vi "LV8_10b.vi"() -> ()   [LabVIEW 2011]
uses:
  <vilib>/imath/engines/lvmath2/RunTimeEngine/ErrorHandling/NIMS_Finalize Error.vi
  <vilib>/imath/engines/lvmath2/RunTimeEngine/NodeEndStatement/NIMS_NodeEndStatement_Output.vi
  <instcachedir>/0/NIMS_NodeEndStatement_Output_53EC0D466D134D7ABD903AC30B43404B.lvgen/NIMS_NodeEndStatement_Output_53EC0D466D134D7ABD903AC30B43404B_000.vi
  <instcachedir>/0/NIMS_NodeEndStatement_Output_53EC0D466D134D7ABD903AC30B43404B.lvgen/NIMS_NodeEndStatement_Output_53EC0D466D134D7ABD903AC30B43404B_005.vi
  <vilib>/imath/engines/lvmath2/RunTimeEngine/RangeToken/NIMS_Range.vi
  <instcachedir>/0/NIMS_Range_0B7635FB69F84E19AA68E7FF959DF37C.lvgen/NIMS_Range_0B7635FB69F84E19AA68E7FF959DF37C_001.vi
  <vilib>/imathl/engines/lvmath/Functions/Error Handling/Create Error.vi
  <vilib>/imath/engines/lvmath2/RunTimeEngine/ArithmeticOperatorToken/NIMS_ArithmeticOperator_times.vi
  <instcachedir>/0/NIMS_ArithmeticOperator_times_3FA9DDB491BD45F6905798C0465C9825.lvgen/NIMS_ArithmeticOperator_times_3FA9DDB491BD45F6905798C0465C9825_000.vi
  <vilib>/imath/engines/lvmath2/RunTimeEngine/BuiltInFunctions/fft/NIMS_fft(GV).vi
  <instcachedir>/0/NIMS_fft(GV)_4C6467FC22F84E4BA42517A07EF978B0.lvgen/NIMS_fft(GV)_4C6467FC22F84E4BA42517A07EF978B0_001.vi
  <vilib>/imath/engines/lvmath2/RunTimeEngine/BuiltInFunctions/abs/NIMS_abs(signed).vi
  <instcachedir>/0/NIMS_abs(signed)_C4FCB8E6058B49B797C7C8D53CA5F6EC.lvgen/NIMS_abs(signed)_C4FCB8E6058B49B797C7C8D53CA5F6EC_006.vi
  <vilib>/imath/engines/lvmath2/RunTimeEngine/BuiltInFunctions/fftshift/NIMS_fftshift(GV).vi
  <instcachedir>/0/NIMS_fftshift(GV)_BD7A7BA9CA6B470B9A9F73A6A3FEEB3E.lvgen/NIMS_fftshift(GV)_BD7A7BA9CA6B470B9A9F73A6A3FEEB3E_001.vi
  <vilib>/imath/engines/lvmath2/RunTimeEngine/ErrorHandling/NIMS_Error From Error Code.vi
  <vilib>/imath/engines/lvmath2/RunTimeEngine/VariableToken/Read/NIMS_Get Elements - RV(_) - Check.vi
  <instcachedir>/0/NIMS_Get Elements - RV(_) - Check_B511B9D8E05044FE80F9F088FE24B20C.lvgen/NIMS_Get Elements - RV(_) - Check_B511B9D8E05044FE80F9F088FE24B20C_000.vi
  <vilib>/imath/engines/lvmath2/RunTimeEngine/BuiltInFunctions/linramp/NIMS_linramp.vi
  <vilib>/imath/engines/lvmath2/RunTimeEngine/ErrorHandling/NIMS_Create Error From Enums.vi
panel:
  in  "stop":bool
  in  "Fmax":dbl(slide)=0.6 scale=0.5..1.0
  in  "Tmax":dbl(slide)=4.0 scale=4.0..10.0
  out "Time Domain":cluster{"f":dbl[], "FX":dbl[]}[](graph)=[{"f"=[-4.0, -3.1666666666666665, -2.333333333333333, -1.5, -0.6666666666666665, 0.16666666666666696, 1.0, 1.833333333333334, 2.666666666666667], "FX"=[0.00013383022576488537, 0.0026509759544301056, 0.026221889093709518, 0.12951759566589174, 0.3194480055223523, 0.3934397161019399, 0.24197072451914337, 0.074311163558993, 0.011395986023797433]}, {"f"=array[2000 elements], "FX"=array[2000 elements]}]
  out "Frequency Domain":cluster{"f":dbl[], "FX":dbl[]}[](graph)=[{"f"=[-0.6, -0.475, -0.35, -0.22499999999999998, -0.09999999999999998, 0.025000000000000022, 0.15000000000000002, 0.275, 0.4], "FX"=[0.0008200746635147077, 0.011635913339555859, 0.08909490952726896, 0.3681379872984424, 0.82086871741554, 0.9877387833616438, 0.6413806259551537, 0.22474751427102416, 0.04249905628536254]}, {"f"=array[2000 elements], "FX"=array[2000 elements]}]
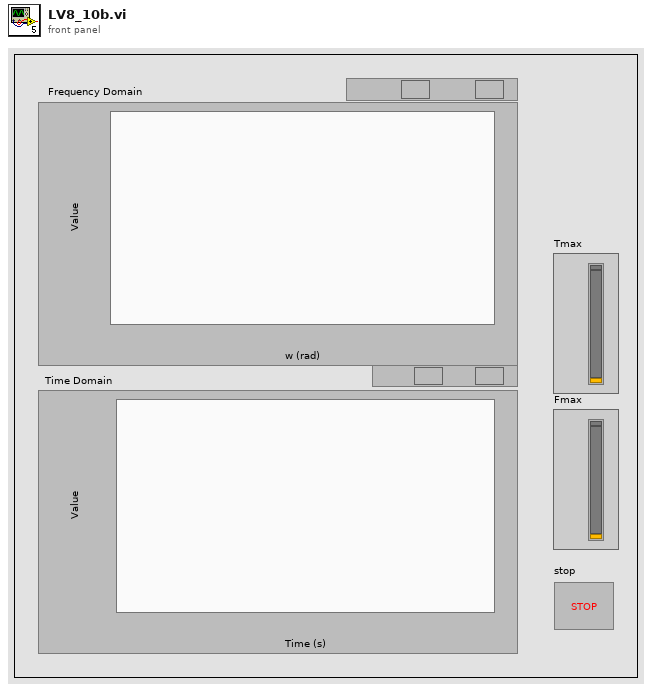
[diagram p1: front panel]
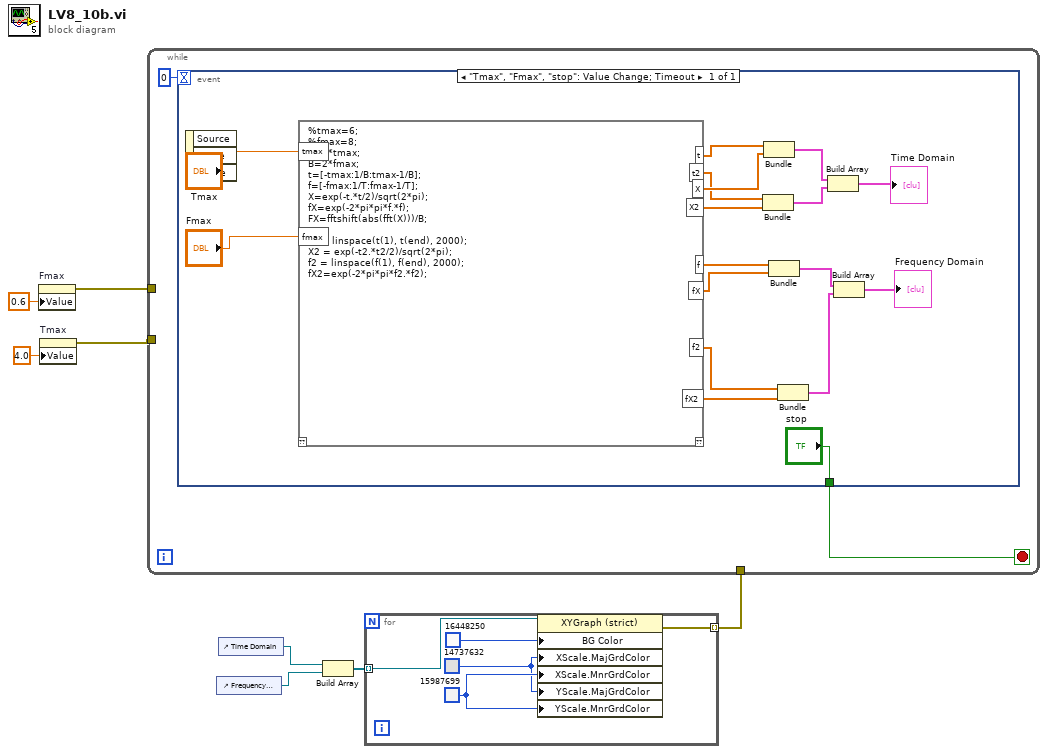
[diagram p0: block diagram]
diagram:
  n1 = property on="Fmax" class="Slide (strict)"("Value"=0.6 ("Fmax")) -> (error out=w6:errorcluster)  [unwired: 2 in, 1 out]
  n2 = property on="Tmax" class="Slide (strict)"("Value"=4.0 ("Tmax")) -> (error out=w5:errorcluster)  [unwired: 2 in, 1 out]
  n3 = control-ref of="Frequency Domain"() -> (w1:refnum<vi>)
  n4 = control-ref of="Time Domain"() -> (w2:refnum<vi>)
  n5 = Build Array(w2, w1) -> (w4:refnum<vi>[])
  n6 = for {
    tunnel: w4 -> [w10] mode=indexing
    tunnel: [w9] -> w3 mode=indexing
    w12 = u32 15987699
    w11 = u32 14737632
    n7 = property class="XYGraph (strict)"(reference=w10, "BG Color"=u32 16448250, "XScale.MajGrdColor"=w11, "XScale.MnrGrdColor"=w12, "YScale.MajGrdColor"=w11, "YScale.MnrGrdColor"=w12) -> (error out=w9:errorcluster)  [unwired: 1 in, 1 out]
  }
  n8 = while {
    tunnel: w6 -> [_]
    tunnel: w5 -> [_]
    tunnel: w3 -> [_]
    stop <- w15 stop-if-true
    n9 = event shown="[0] \"Tmax\", \"Fmax\", \"stop\": Value Change;  Timeout" {
      selector: _ -> [_]
      dyn-events: _ -> [_]
      timeout: 0 -> [_]
      tunnel: ["stop"] -> w15
      event "Tmax", "Fmax", "stop": Value Change; Timeout {
        n10 = event-data() -> ()  [unwired: 1 in, 3 out]
        n11 = mathscript code="%tmax=6;\n%fmax=8;\nT=2*tmax;\nB=2*fmax;\nt=[-tmax:1/B:tmax-1/B];\nf=[-fmax:1/T:fmax-1/T];\nX=exp(-t.*t/2)/sqrt(2*pi);\nfX=exp(-2*pi*pi*f.*f);\nFX=fftshift(abs(fft(X)))/B;\n\nt2 = linspace(t(1), t(end), 2000);\nX2 = exp(-t2.*t2/2)/sqrt(2*pi);\nf2 = linspace(f(1), f(end), 2000);\nfX2=exp(-2*pi*pi*f2.*f2);"("tmax"="Tmax", "fmax"="Fmax") -> ("f"=w31:dbl[], "fX"=w32:dbl[], "fX2"=w26:dbl[], "f2"=w27:dbl[], "t"=w25:dbl[], "t2"=w23:dbl[], "X"=w24:cdb[], "X2"=w22:cdb[])  [unwired: 1 in, 1 out]
        n12 = Bundle("t2"=w23, "X2"=w22) -> (w20:cluster{"t2":dbl[], "X2":cdb[]})  [unwired: 1 in]
        n13 = Bundle("t"=w25, "X"=w24) -> (w21:cluster{"t":dbl[], "X":cdb[]})  [unwired: 1 in]
        n14 = Bundle("f"=w31, "fX"=w32) -> (w30:cluster{"f":dbl[], "fX":dbl[]})  [unwired: 1 in]
        n15 = Bundle("f2"=w27, "fX2"=w26) -> (w29:cluster{"f2":dbl[], "fX2":dbl[]})  [unwired: 1 in]
        n16 = Build Array(w21, w20) -> (→"Time Domain":cluster{"t2":dbl[], "X2":cdb[]}[])
        n17 = Build Array(w30, w29) -> (→"Frequency Domain":cluster{"f2":dbl[], "fX2":dbl[]}[])
      }
    }
  }
